vi "List Managers.vi"(10 "Include Cache? (F)":bool, 11 "SMOConfigManager.Cache in":refnum<class "ConfigManager.Cache.lvclass">) -> (2 "List":refnum<class "ConfigManager.lvclass">[](array[class]), 3 "SMOConfigManager.Cache out":refnum<class "ConfigManager.Cache.lvclass">)   [LabVIEW 2013, in "SMOConfig.lvlib" / "ConfigManager.Cache.lvclass"]
uses:
  ConfigManager.Cache.lvclass
  Manager/ConfigManager.lvclass
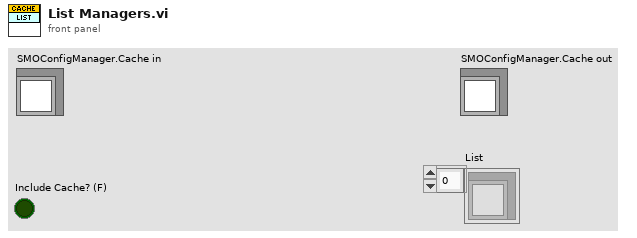
[diagram p1: front panel]
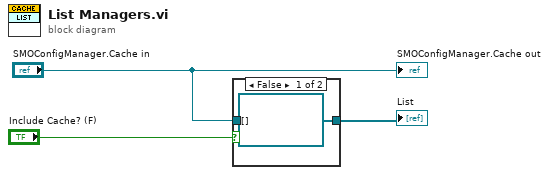
[diagram p0: block diagram]
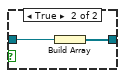
[diagram p2: hidden frame]
diagram:
  n1 = case shown="False" "Include Cache? (F)" {
    tunnel: "SMOConfigManager.Cache in" -> [_ w6]
    tunnel: [refnum<class "ConfigManager.lvclass">[] [] w5] -> w2
    frame False {
    }
    frame True {
      n2 = Build Array(w6) -> (w5:refnum<class "ConfigManager.Cache.lvclass">[])
    }
  }
  "List" <- w2
  "SMOConfigManager.Cache out" <- "SMOConfigManager.Cache in"
